vi "Replace MNU Files.vi"(5 "display name":string, 6 "Palette 2 Source Path":path=path "C:/Program Files (x86)/National Instruments/LabVIEW 2010/user.lib/_FPGA Interface Advanced Tools/FPGA Interface By TypeDefs/FIFO Utility.mnu", 7 "Palette 1 Source Path":path=path "C:/Program Files (x86)/National Instruments/LabVIEW 2010/user.lib/_FPGA Interface Advanced Tools/FPGA Interface By TypeDefs/dir.mnu", 8 "error in":errorcluster, 9 "Palette 2 Destination Path":path=path "C:/Users/mlyons/Desktop/test/FIFO Utility.mnu", 10 "Palette 1 Destination Path":path=path "C:/Users/mlyons/Desktop/test/dir.mnu", 11 "LVClass path":path=path "C:/Users/mlyons/Desktop/test/iLoveArina.lvclass") -> (0 "error out":errorcluster)   [LabVIEW 2010]
uses:
  <vilib>/Palette API/Palette Menu/Public Type Define/Palette type.ctl
  <vilib>/Utility/sysdir.llb/System Directory Type.ctl
  <vilib>/Palette API/Palette Menu/Palette Menu.lvlib
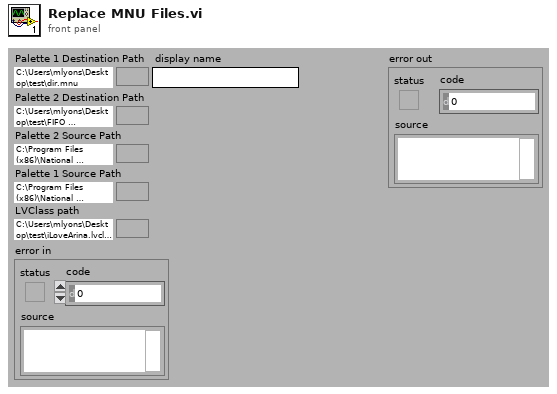
[diagram p1: front panel]
types:
  T1 = typedef "System Directory Type.ctl" = i32
  T2 = typedef "Palette Menu.lvlib/Palette type.ctl" = i32
  T3 = typedef "Palette Menu.lvlib/Palette Data.ctl" = cluster{"display name":string, "view format":T4, "palette width":i16, "items":T5, "256 color icon":picture, "B&W color icon":picture, "help information":T7, "palette description":string, "synchronize information":T8}
  T4 = typedef "Palette Menu.lvlib/View Format.ctl" = u16
  T5 = typedef "Palette Menu.lvlib/Items.ctl" = T6[]
  T6 = typedef "Palette Menu.lvlib/Item.ctl" = cluster{"item path":path, "library path (.lvlib)":path, "use default lvlib palette":bool, "short name":string, "place VI contents":bool, "hide synchronized item":bool, "reserve spot for synch item":bool, "configure when placing VI contents":bool}
  T7 = typedef "Palette Menu.lvlib/Help Info.ctl" = cluster{"help tag":string, "help file path ":path}
  T8 = typedef "Palette Menu.lvlib/Synchronize Info.ctl" = cluster{"synchronize with directory":bool, "synchronize directory path":path}
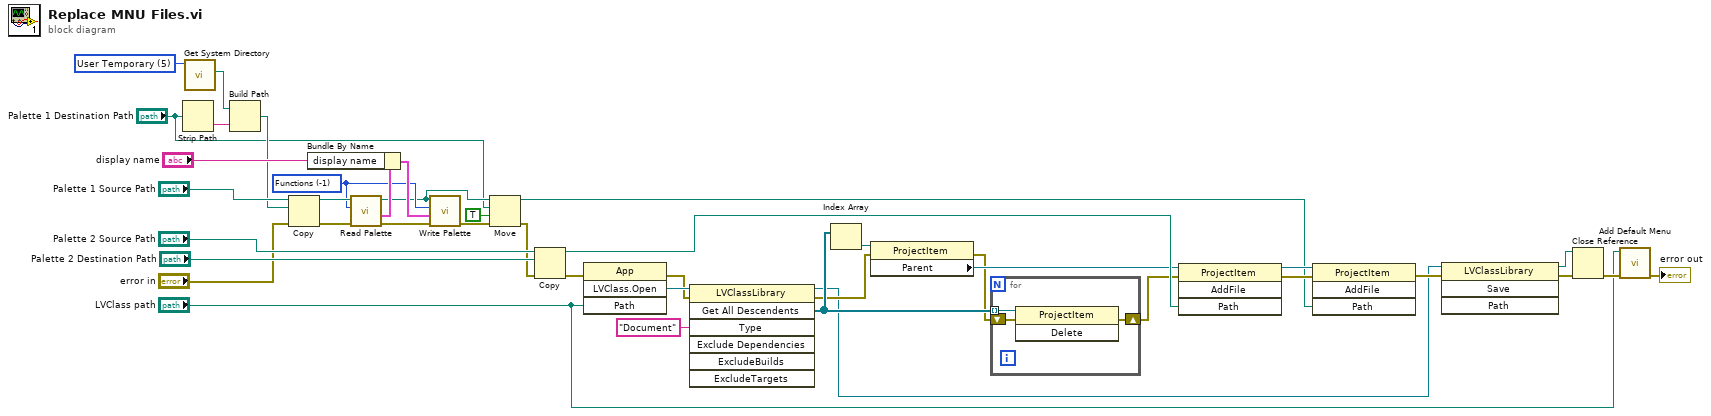
[diagram p0: block diagram]
diagram:
  w10 = T1 5 items=["User Home"=0, "User Desktop"=1, "User Documents"=2, "User Application Data"=3, "User Preferences"=4, "User Temporary"=5, "Public Documents"=6, "Public Application Data"=7, "Public Preferences"=8, "Public Cache"=13, "System Core Libraries"=9, "System Installed Libraries"=10, "Application Files"=11, "Boot Volume Root"=12] ("system directory type")
  w12 = T2 -1 items=["Functions"=-1, "Controls"=-2] ("palette type")
  n1 = Strip Path(path="Palette 1 Destination Path") -> (name=w8:string)  [unwired: 1 out]
  n2 = call <vilib>:"Get System Directory.vi"("system directory type"=w10) -> ("system directory"=w9:path)  [unwired: 10 in]
  n3 = Build Path(base path=w9, name or relative path=w8) -> (appended path=w7:path)
  n4 = Copy(8:"error in", 10:w7, 11:"Palette 1 Source Path") -> (0:w14:errorcluster, 3:w17:path)  [unwired: 2 in, 1 out]
  n5 = call <vilib>:"Read Palette.vi"("error in (no error)"=w14, "palette type"=w12, "palette path"=w17) -> ("error out"=w15:errorcluster, "palette data"=w16:T3, "duplicate palette path"=w5:path)  [unwired: 6 in]
  n6 = Bundle By Name(cluster=w16, "display name"="display name") -> (w13:T3)
  n7 = call <vilib>:"Write Palette.vi"("error in (no error)"=w15, "palette data"=w13, "palette type"=w12, "palette path"=w5) -> ("error out"=w6:errorcluster)  [unwired: 7 in]
  n8 = Move(source path=w5, error in=w6, 9:TRUE ("overwrite (F)"), 10:"Palette 1 Destination Path") -> (error out=w3:errorcluster, 3:w1:path)  [unwired: 1 in, 1 out]
  n9 = Copy(8:w3, 10:"Palette 2 Destination Path", 11:"Palette 2 Source Path") -> (0:w41:errorcluster, 3:w36:path)  [unwired: 2 in, 1 out]
  n10 = invoke class="App" method="LVClass.Open"(error in=w41, "Path"="LVClass path") -> (error out=w35:errorcluster, "LVClass.Open"=w40:refnum<vi>)  [unwired: 2 in, 2 out]
  n11 = invoke class="LVClassLibrary" method="Get All Descendents"(reference=w40, error in=w35, "Type"="Document") -> (reference out=w24:refnum<vi>, error out=w31:errorcluster, "All Descendents"=w33:refnum<vi>[])  [unwired: 4 in, 4 out]
  n12 = Index Array(array=w33) -> (element=w32:refnum<vi>)  [unwired: 1 in]
  n13 = property class="ProjectItem"(reference=w32, error in=w31) -> (error out=w27:errorcluster, "Parent"=w30:refnum<vi>)  [unwired: 1 out]
  n14 = for {
    tunnel: w33 -> [w44] mode=indexing
    shift-right: [w42] -> w26
    shift-left: w27 -> [w43]
    n15 = invoke class="ProjectItem" method="Delete"(reference=w44, error in=w43) -> (error out=w42:errorcluster)  [unwired: 1 in, 2 out]
  }
  n16 = invoke class="ProjectItem" method="AddFile"(reference=w30, error in=w26, "Path"=w36) -> (reference out=w29:refnum<vi>, error out=w28:errorcluster)  [unwired: 1 in, 2 out]
  n17 = invoke class="ProjectItem" method="AddFile"(reference=w29, error in=w28, "Path"=w1) -> (error out=w25:errorcluster)  [unwired: 1 in, 3 out]
  n18 = invoke class="LVClassLibrary" method="Save"(reference=w24, error in=w25) -> (reference out=w22:refnum<vi>, error out=w23:errorcluster)  [unwired: 2 in, 2 out]
  n19 = Close Reference(reference=w22, error in (no error)=w23) -> (error out=w21:errorcluster)
  n20 = call "Add Default Menu.vi"("error in"=w21, "Path"="LVClass path") -> ("error out"=→"error out":errorcluster)  [unwired: 9 in]
